vi "Paint_Tracks_Before-After-3.vi"(0 "[IN] Frame":T2, 1 "[IN] Destina\ntion Image":T2, 2 "[IN] AVI Refnum":T3, 3 "[IN] # channel":u8, 5 "[IN] Testing Frame":u32 min=24 max=58, 7 "[IN] Tracks group":i32 min=0 max=258, 9 "[IN] Grouped Tracks":T4(array[cluster]), 10 "Keep Nega-\ntive Values?":bool, 11 "error IN":errorcluster, 12 "[IN] Filtering Settings":T1, 13 "[IN] Delete Tracs":bool, 14 "[IN] Additional Index":i32) -> (4 "[OUT] Image with\nDisplacements":T2, 15 "error OUT":errorcluster)   [LabVIEW 2013]
uses:
  <vilib>/vision/Image Controls.llb/IMAQ Image.ctl
  <vilib>/vision/Avi.llb/IMAQ AVI2 Refnum.ctl
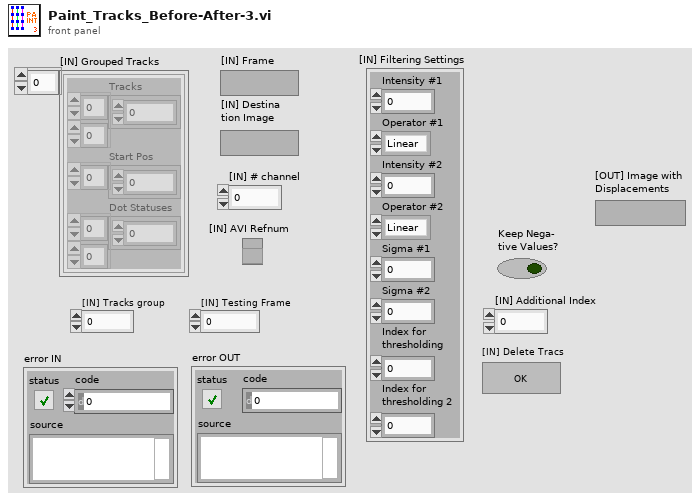
[diagram p1: front panel]
types:
  T1 = cluster{"Intensity #1":sgl, "Operator #1":enum32{"Linear", "Log", "Exp", "Square", "Square root", "Power X", "Power 1/X"}, "Intensity #2":sgl, "Operator #2":enum32{"Linear", "Log", "Exp", "Square", "Square root", "Power X", "Power 1/X"}, "Sigma #1":dbl, "Sigma #2":dbl, "Index for \nthresholding":u8, "Index for \nthresholding 2":u8}
  T2 = typedef "IMAQ Image.ctl" = refnum<image>
  T3 = typedef "IMAQ AVI2 Refnum.ctl" = refnum<k20>
  T4 = cluster{"Tracks":dbl[][], "Start Pos":i32[], "Dot Statuses":i16[][]}[]
  T5 = cluster{"Tracks":dbl[][], "Start Pos":i32[], "Dot Statuses":i16[][]}
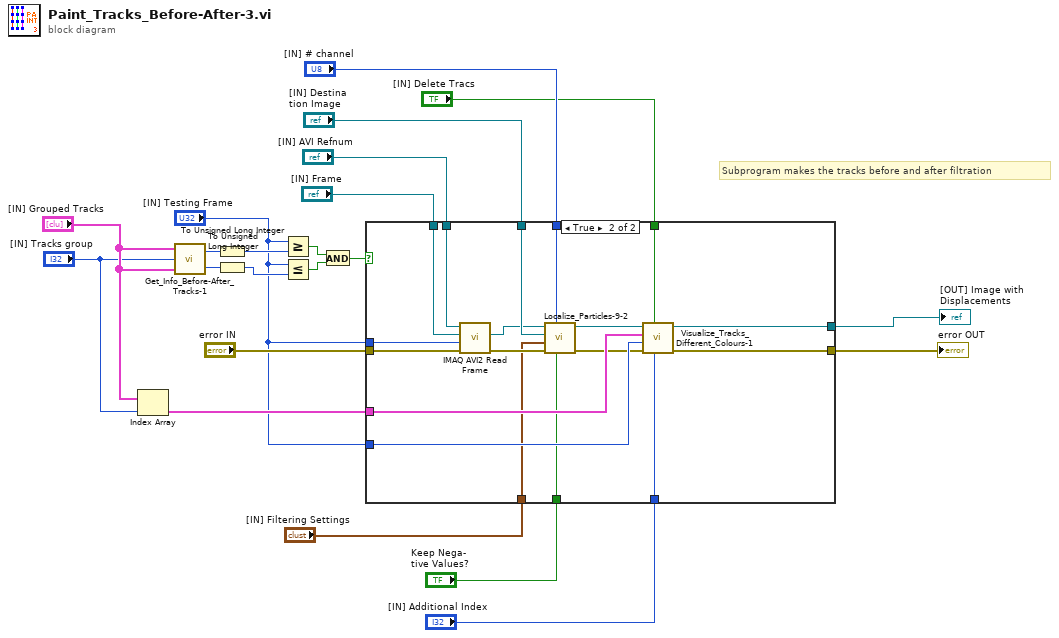
[diagram p0: block diagram]
diagram:
  # "Subprogram makes the tracks before and after filtration"
  n1 = Index Array(array="[IN] Grouped Tracks", index="[IN] Tracks group") -> (element=w9:T5)
  n2 = call "Get_Info_Before-After_Tracks-1.vi"("[IN] After Tracks"="[IN] Grouped Tracks", "[IN] Tracks group"="[IN] Tracks group", "[IN] Before Tracks"="[IN] Grouped Tracks") -> ("Maximal Frame\n(finish point all\ntracks)"=w20:i32, "[OUT] Min Start Pos"=w22:i32)
  n3 = To Unsigned Long Integer(number=w22) -> (unsigned 32bit integer=w21:u32)
  n4 = To Unsigned Long Integer(number=w20) -> (unsigned 32bit integer=w19:u32)
  n5 = Greater Or Equal?(x="[IN] Testing Frame", y=w21) -> (x >= y?=w18:bool)
  n6 = Less Or Equal?(x="[IN] Testing Frame", y=w19) -> (x <= y?=w17:bool)
  n7 = And(x=w18, y=w17) -> (x .and. y?=w16:bool)
  n8 = case shown="True" w16 {
    tunnel: "error IN" -> [w23 w42]
    tunnel: "[IN] AVI Refnum" -> [_ w41]
    tunnel: "[IN] Frame" -> [_ w40]
    tunnel: "[IN] Testing Frame" -> [_ w39]
    tunnel: "[IN] # channel" -> [_ w28]
    tunnel: w9 -> [_ w38]
    tunnel: "[IN] Destina\ntion Image" -> [w24 w30]
    tunnel: "[IN] Testing Frame" -> [_ w37]
    tunnel: [w24 w36] -> w5
    tunnel: [w23 w35] -> w6
    tunnel: "[IN] Delete Tracs" -> [_ w34]
    tunnel: "[IN] Additional Index" -> [_ w33]
    tunnel: "[IN] Filtering Settings" -> [_ w31]
    tunnel: "Keep Nega-\ntive Values?" -> [_ w25]
    frame False {
    }
    frame True {
      n9 = call "IMAQ AVI2 Read Frame"("error in (no error)"=w42, "Frame Number"=w39, "Image"=w40, "AVI Refnum"=w41) -> ("error out"=w32:errorcluster, "Image Out"=w29:T2)  [unwired: 5 in, 1 out]
      n10 = call "Localize_Particles-9-2.vi"("Keep Nega-\ntive Values?"=w25, "# channel"=w28, "error IN"=w32, "[IN] Filtering Settings"=w31, "[IN] Destination Image"=w30, "[IN] Frame"=w29) -> ("error OUT"=w26:errorcluster, "[OUT] LoG Processed Image"=w27:T2)  [unwired: 1 in, 1 out]
      n11 = call "Visualize_Tracks_Different_Colours-1.vi"("[IN] Additional Index"=w33, "[IN] Delete Tracs"=w34, "error IN"=w26, "[IN] Testing Frame"=w37, "[IN] Tracks"=w38, "[IN] LoG Pro-\ncessed Image"=w27) -> ("error OUT"=w35:errorcluster, "[OUT] Image with\nDisplacements"=w36:T2)  [unwired: 2 in]
    }
  }
  "error OUT" <- w6
  "[OUT] Image with\nDisplacements" <- w5
